vi "SetSelectRowColor(Tab).vi"(9 "OthersRow":u32(colorbox)=16448250, 10 "SelectRow":u32(colorbox)=12369084, 11 "Table输入":refnum<vi>) -> ()   [LabVIEW 2018]
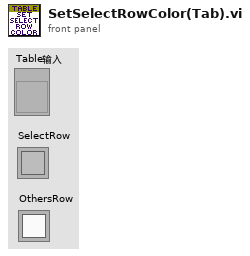
[diagram p1: front panel]
types:
  T1 = typedef "LVRowAndColumnTypeDef.ctl" = cluster{"Row":i32, "Column":i32}
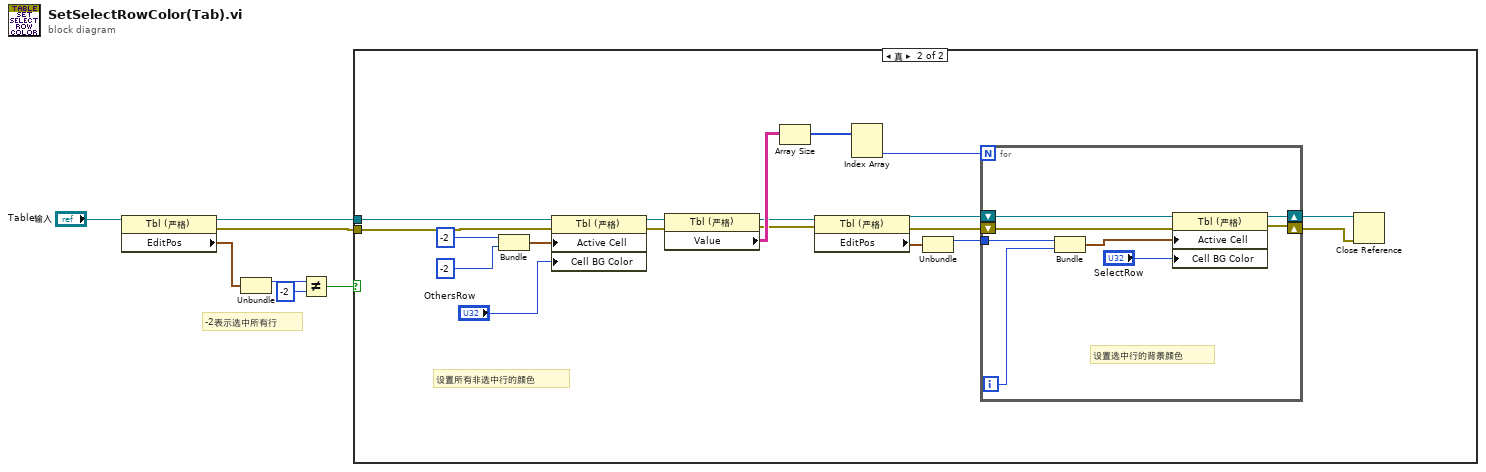
[diagram p0: block diagram]
diagram:
  # "-2表示选中所有行"
  n1 = property class="Tbl (严格)"(reference="Table输入") -> (reference out=w6:refnum<vi>, error out=w1:errorcluster, "EditPos"=w5:T1)  [unwired: 1 in]
  n2 = Unbundle(w5) -> ("Row"=w4:i32)  [unwired: 1 out]
  n3 = Not Equal?(x=w4, y=-2) -> (x != y?=w2:bool)
  n4 = case shown="真" w2 {
    tunnel: w6 -> [_ w16]
    tunnel: w1 -> [_ w15]
    frame False {
    }
    frame True {
      # "设置所有非选中行的颜色"
      n5 = Bundle(-2, -2) -> (w19:cluster{i32, i32})  [unwired: 1 in]
      n6 = property class="Tbl (严格)"(reference=w16, error in=w15, "Active Cell"=w19, "Cell BG Color"="OthersRow") -> (reference out=w14:refnum<vi>, error out=w13:errorcluster)
      n7 = property class="Tbl (严格)"(reference=w14, error in=w13) -> (reference out=w9:refnum<vi>, error out=w8:errorcluster, "Value"=w12:string[][])
      n8 = Array Size(array=w12) -> (size(s)=w11:i32[])
      n9 = property class="Tbl (严格)"(reference=w9, error in=w8) -> (reference out=w25:refnum<vi>, error out=w24:errorcluster, "EditPos"=w26:T1)
      n10 = Index Array(array=w11) -> (element #2=w10:i32)  [unwired: 2 in, 1 out]
      n11 = Unbundle(w26) -> ("Row"=w23:i32)  [unwired: 1 out]
      n12 = for {
        N: w10 -> [_]
        tunnel: w23 -> [w31]
        shift-right: [w30] -> w22
        shift-left: w25 -> [w34]
        shift-right: [w29] -> w21
        shift-left: w24 -> [w33]
        i -> [w28]
        # "设置选中行的背景颜色"
        n13 = Bundle("Row"=w31, w28) -> (w32:cluster{"Row":i32, i32})  [unwired: 1 in]
        n14 = property class="Tbl (严格)"(reference=w34, error in=w33, "Active Cell"=w32, "Cell BG Color"="SelectRow") -> (reference out=w30:refnum<vi>, error out=w29:errorcluster)
      }
      n15 = Close Reference(reference=w22, error in (no error)=w21) -> ()  [unwired: 1 out]
    }
  }
